vi "Find Center Setup_01282025.vi"(0 "Carrier Tray":T1, 1 "Tray Number":dbl format="%#_13g", 2 "Position":i32, 3 "Assembly Type":string) -> (7 "Assembly Tray Out":T1)   [LabVIEW 2021, in "Assembly Tray.lvclass"]
uses:
  Assembly Tray.lvclass
  Find Tray.ctl
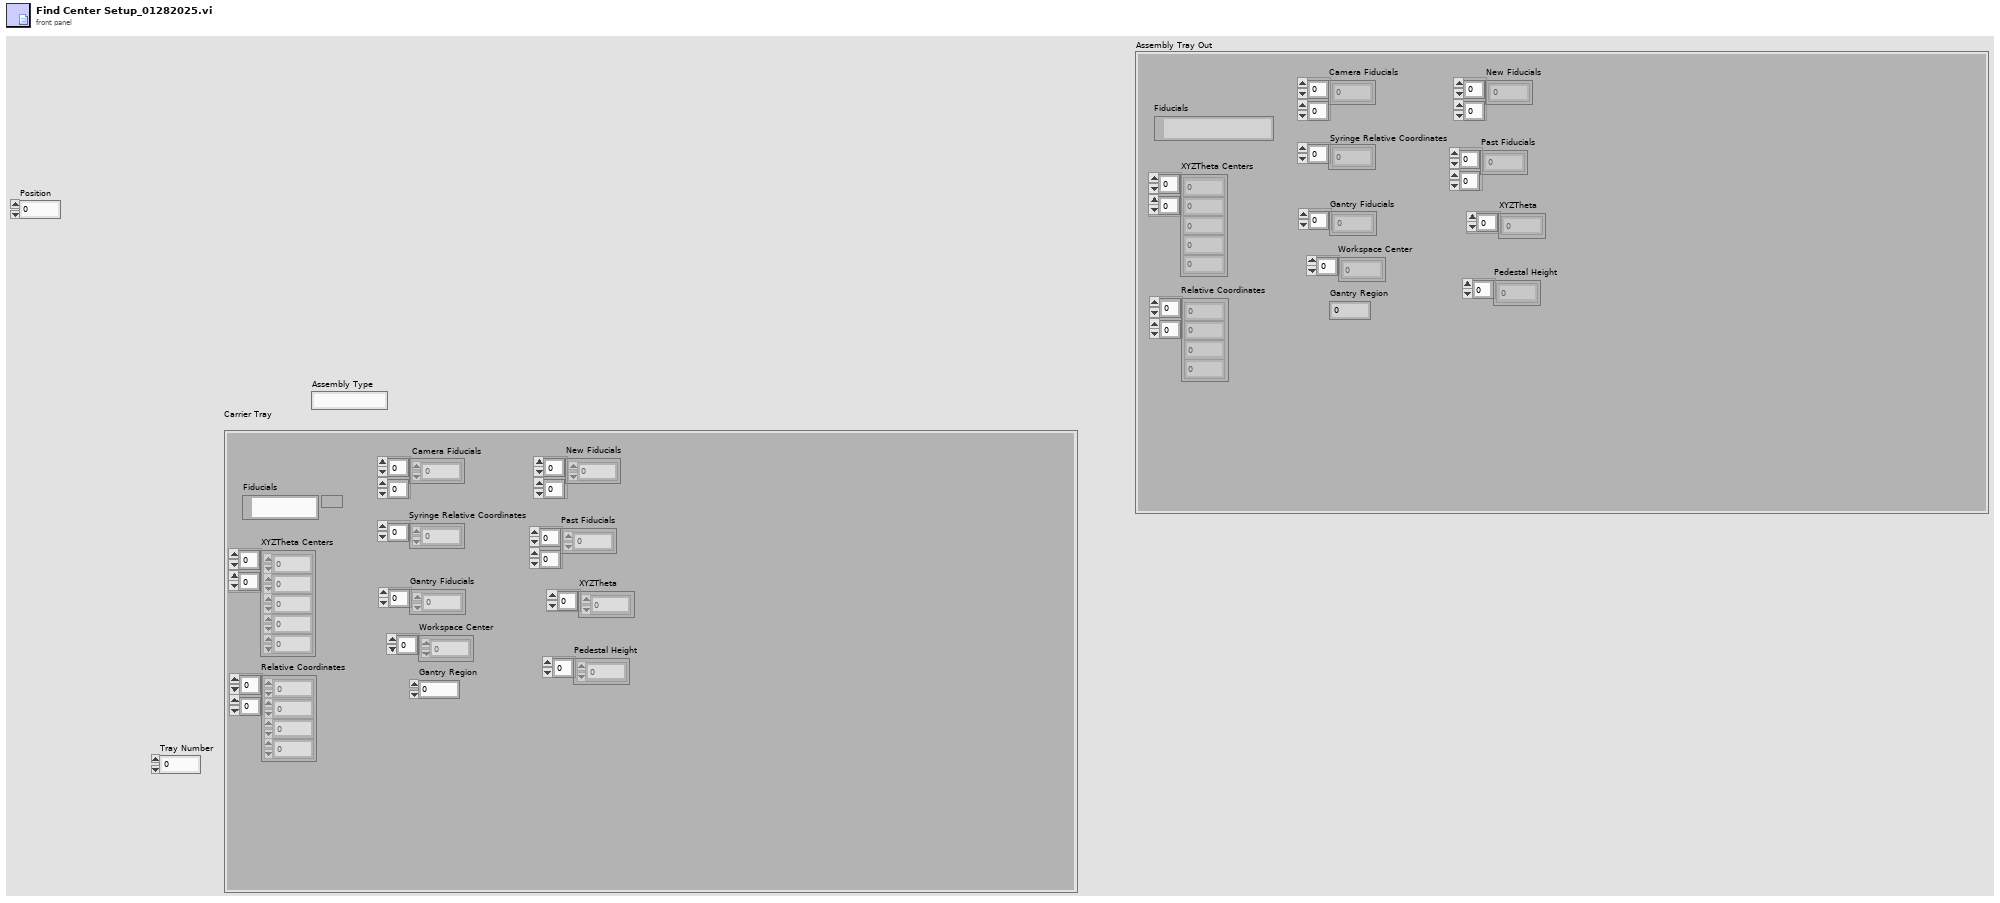
[diagram p1: front panel]
types:
  T1 = typedef "Assembly Tray.lvclass/Find Tray.ctl" = cluster{"Gantry Fiducials":dbl[], "Relative Coordinates":dbl[][], "Camera Fiducials":dbl[][], "XYZTheta Centers":dbl[][], "Workspace Center":dbl[], "Syringe Relative Coordinates":dbl[], "Gantry Region":dbl, "Fiducials":path, "New Fiducials":dbl[][], "Past Fiducials":dbl[][], "XYZTheta":dbl[], "Pedestal Height":dbl[]}
  T2 = typedef "File Paths.ctl" = cluster{"Glue Pattern Folder":path, "Carrier Tray Folder":path, "Pick Up Tool Fixture Folder":path, "Components Folder":path, "Bellows Tool Offset.txt":path, "Pick Up Tool Offset.txt":path, "Dispense Tip Offset.txt":path, "Log Files":path, "Gantry Assembly Map.txt":path, "Syringe and offset map.txt":path, "Controllers Folder":path, "Local dbase config":path}
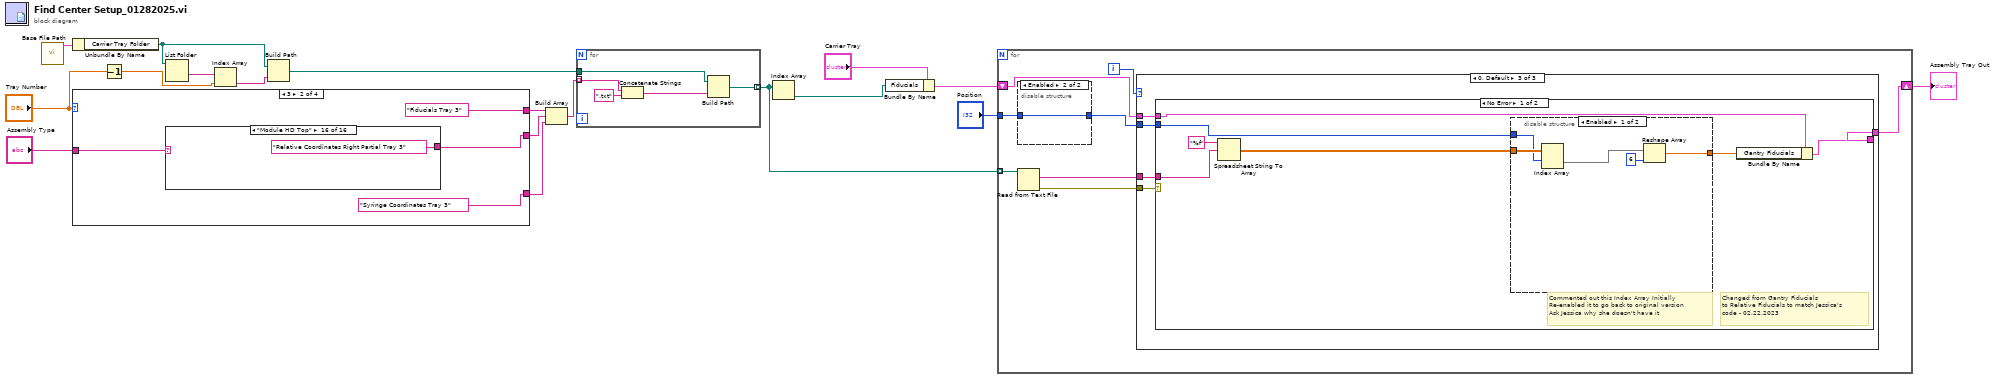
[diagram p0: block diagram]
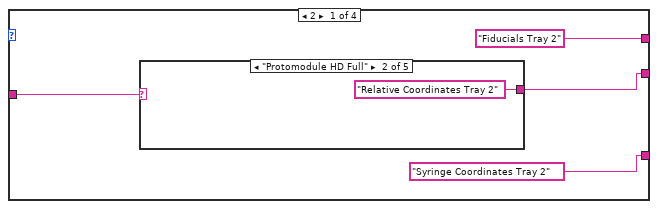
[diagram p2: hidden frame]
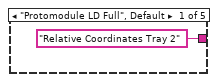
[diagram p3: hidden frame]
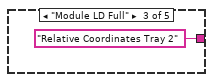
[diagram p4: hidden frame]
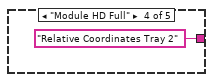
[diagram p5: hidden frame]
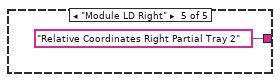
[diagram p6: hidden frame]
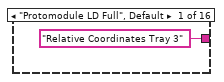
[diagram p7: hidden frame]
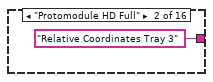
[diagram p8: hidden frame]
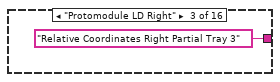
[diagram p9: hidden frame]
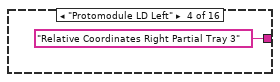
[diagram p10: hidden frame]
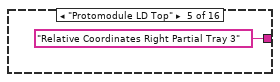
[diagram p11: hidden frame]
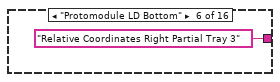
[diagram p12: hidden frame]
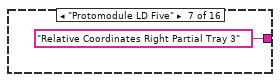
[diagram p13: hidden frame]
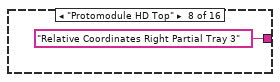
[diagram p14: hidden frame]
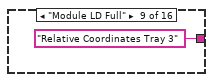
[diagram p15: hidden frame]
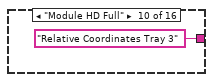
[diagram p16: hidden frame]
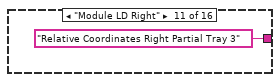
[diagram p17: hidden frame]
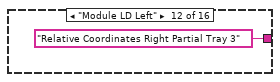
[diagram p18: hidden frame]
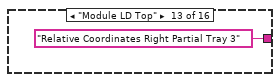
[diagram p19: hidden frame]
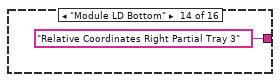
[diagram p20: hidden frame]
diagram:
  n1 = call "Base File Path.vi"() -> ("Paths Out"=w13:T2)  [unwired: 11 in]
  n2 = Unbundle By Name(w13) -> ("Carrier Tray Folder"=w6:path)
  n3 = case shown="3" "Tray Number" {
    tunnel: [w21 w30 w50 w63] -> w9
    tunnel: "Assembly Type" -> [w22 w31 w51 w62]
    tunnel: ["Fiducials Tray 2" ("format string") "Fiducials Tray 3" ("format string") "Fiducials Tray 3" ("format string") "Fiducials" ("format string")] -> w4
    tunnel: ["Syringe Coordinates Tray 2" ("element") "Syringe Coordinates Tray 3" ("element") "Syringe Coordinates Tray 3" ("element") "Syringe Coordinates" ("element")] -> w3
    frame 2 {
      n4 = case shown="\"Protomodule HD Full\"" w22 {
        tunnel: ["Relative Coordinates Tray 2" ("format string") "Relative Coordinates Tray 2" ("format string") "Relative Coordinates Tray 2" ("format string") "Relative Coordinates Tray 2" ("format string") "Relative Coordinates Right Partial Tray 2" ("format string")] -> w21
        frame "Protomodule LD Full", Default {
        }
        frame "Protomodule HD Full" {
        }
        frame "Module LD Full" {
        }
        frame "Module HD Full" {
        }
        frame "Module LD Right" {
        }
      }
    }
    frame 3 {
      n5 = case shown="\"Module HD Top\"" w31 {
        tunnel: ["Relative Coordinates Tray 3" ("format string") "Relative Coordinates Tray 3" ("format string") "Relative Coordinates Right Partial Tray 3" ("format string") "Relative Coordinates Right Partial Tray 3" ("format string") "Relative Coordinates Right Partial Tray 3" ("format string") "Relative Coordinates Right Partial Tray 3" ("format string") "Relative Coordinates Right Partial Tray 3" ("format string") "Relative Coordinates Right Partial Tray 3" ("format string") "Relative Coordinates Tray 3" ("format string") "Relative Coordinates Tray 3" ("format string") "Relative Coordinates Right Partial Tray 3" ("format string") "Relative Coordinates Right Partial Tray 3" ("format string") "Relative Coordinates Right Partial Tray 3" ("format string") "Relative Coordinates Right Partial Tray 3" ("format string") "Relative Coordinates Right Partial Tray 3" ("format string") "Relative Coordinates Right Partial Tray 3" ("format string")] -> w30
        frame "Protomodule LD Full", Default {
        }
        frame "Protomodule HD Full" {
        }
        frame "Protomodule LD Right" {
        }
        frame "Protomodule LD Left" {
        }
        frame "Protomodule LD Top" {
        }
        frame "Protomodule LD Bottom" {
        }
        frame "Protomodule LD Five" {
        }
        frame "Protomodule HD Top" {
        }
        frame "Module LD Full" {
        }
        frame "Module HD Full" {
        }
        frame "Module LD Right" {
        }
        frame "Module LD Left" {
        }
        frame "Module LD Top" {
        }
        frame "Module LD Bottom" {
        }
        frame "Module LD Five" {
        }
        frame "Module HD Top" {
        }
      }
    }
    frame 4 {
      n6 = case shown="\"Module LD Right\"" w51 {
        tunnel: ["Relative Coordinates Tray 3" ("format string") "Relative Coordinates Tray 3" ("format string") "Relative Coordinates Right Partial Tray 3" ("format string") "Relative Coordinates Right Partial Tray 3" ("format string") "Relative Coordinates Tray 3" ("format string") "Relative Coordinates Tray 3" ("format string") "Relative Coordinates Right Partial Tray 4" ("format string") "Relative Coordinates Right Partial Tray 3" ("format string")] -> w50
        frame "Protomodule LD Full", Default {
        }
        frame "Protomodule HD Full" {
        }
        frame "Protomodule LD Right" {
        }
        frame "Protomodule LD Left" {
        }
        frame "Module LD Full" {
        }
        frame "Module HD Full" {
        }
        frame "Module LD Right" {
        }
        frame "Module LD Left" {
        }
      }
    }
    frame 1, Default {
      n7 = case shown="\"Module LD Right\"" w62 {
        tunnel: ["Relative Coordinates" ("format string") "Relative Coordinates" ("format string") "Relative Coordinates Right Partial" ("format string")] -> w63
        frame "Protomodule LD Full", Default {
        }
        frame "Module LD Full" {
        }
        frame "Module LD Right" {
        }
      }
    }
  }
  n8 = Decrement(x="Tray Number") -> (x-1=w11:dbl)
  n9 = List Folder(path=w6) -> (folder names=w15:string[])  [unwired: 3 in, 3 out]
  n10 = Index Array "Index Array"(array=w15, index=w11) -> (element=w14:string)
  n11 = Build Path(base path=w6, name or relative path=w14) -> (appended path=w7:path)
  n12 = Build Array(w4, w9, w3) -> (w16:string[])
  n13 = for {
    tunnel: w16 -> [w70] mode=indexing
    tunnel: w7 -> [w71]
    tunnel: [w67] -> w8 mode=indexing
    n14 = Concatenate Strings "Concatenate Strings"(w70, ".txt" ("string")) -> (w68:string)
    n15 = Build Path(base path=w71, name or relative path=w68) -> (appended path=w67:path)
  }
  n16 = Index Array "Index Array"(array=w8) -> (element=w17:path)  [unwired: 1 in]
  n17 = Bundle By Name "Bundle By Name"(cluster="Carrier Tray", "Fiducials"=w17) -> (w18:T1)
  n18 = for {
    tunnel: w8 -> [w78] mode=indexing
    shift-right: [w74] -> w12
    shift-left: w18 -> [w75]
    tunnel: "Position" -> [w73]
    i -> [w76]
    n19 = disable-structure shown="Enabled" {
      disable-tunnel: w73 -> [w81 w83]
      disable-tunnel: [w80 w83] -> w72
      frame Disabled {
        n20 = Add(x=1, y=w81) -> (x+y=w80:i32)
      }
      frame Enabled {
      }
    }
    n21 = Read from Text File(file (use dialog)=w78) -> (text=w79:string, error out=w77:errorcluster)  [unwired: 3 in, 2 out]
    n22 = case shown="0, Default" w76 {
      tunnel: w79 -> [w86 w101 w117]
      tunnel: w77 -> [w87 w102 w116]
      tunnel: w75 -> [w85 w103 w115]
      tunnel: [w84 w100 w114] -> w74
      tunnel: w72 -> [_ _ w113]
      frame 1 {
        n23 = case shown="No Error" w87 {
          tunnel: w86 -> [w94 _]
          tunnel: [w92 w97] -> w84
          tunnel: w85 -> [w93 w97]
          frame No Error {
            n24 = Spreadsheet String To Array(format string="%f", spreadsheet string=w94, array type (2D Dbl)=dbl[][] []) -> (array=w91:dbl[][])  [unwired: 1 in]
            n25 = Array Subset(array=w91, index (row)=1 ("length"), index (col)=1 ("index (row)")) -> (w90:dbl[][])  [unwired: 2 in]
            n26 = Bundle By Name(cluster=w93, "Relative Coordinates"=w90) -> (w92:T1)
          }
          frame Error {
            n27 = One Button Dialog(message="Relative Coordinates Not Found") -> (true=w98:bool)  [unwired: 1 in]
            n28 = Stop(stop? (T)=w98) -> ()
          }
        }
      }
      frame 2 {
        n29 = case shown="No Error" w102 {
          tunnel: w101 -> [w107 _]
          tunnel: [w105 w110] -> w100
          tunnel: w103 -> [w106 w110]
          frame No Error {
            n30 = Spreadsheet String To Array(format string="%f", spreadsheet string=w107, array type (2D Dbl)=dbl[] []) -> (array=w104:dbl[])  [unwired: 1 in]
            n31 = Bundle By Name(cluster=w106, "Syringe Relative Coordinates"=w104) -> (w105:T1)
          }
          frame Error {
            n32 = One Button Dialog(message="Syringe Coordinates Not Found") -> (true=w111:bool)  [unwired: 1 in]
            n33 = Stop(stop? (T)=w111) -> ()
          }
        }
      }
      frame 0, Default {
        n34 = case shown="No Error" w116 {
          tunnel: w117 -> [w123 _]
          tunnel: w115 -> [w121 w134]
          tunnel: [w122 w134] -> w114
          tunnel: w113 -> [w118 _]
          frame No Error {
            # "Commented out this Index Array Initially\nRe-enabled it to go back to original version\nAsk Jessica why she doesn't have it"
            # "Changed from Gantry Fiducials\nto Relative Fiducials to match Jessica's \ncode - 02.22.2023"
            n35 = Spreadsheet String To Array(format string="%f", spreadsheet string=w123) -> (array=w119:dbl[][])  [unwired: 2 in]
            n36 = disable-structure shown="Enabled" {
              disable-tunnel: [w129 w130] -> w120
              disable-tunnel: w119 -> [w128 w133]
              disable-tunnel: w118 -> [w125 _]
              frame Enabled {
                n37 = Index Array "Index Array"(array=w128, index (row)=w125) -> (element=w127:dbl[])  [unwired: 1 in]
                n38 = Reshape Array "Reshape Array"(w127, 6 ("dimension size")) -> (w129:dbl[])
              }
              frame Disabled {
                n39 = Delete From Array "Delete From Array"() -> ()  [unwired: 3 in, 2 out]
                n40 = Reshape Array "Reshape Array"(w133, 1 ("dimension size"), 1 ("dimension size")) -> (w130:dbl[][])
              }
            }
            n41 = Bundle By Name "Bundle By Name"(cluster=w121, "Gantry Fiducials"=w120) -> (w122:T1)
          }
          frame Error {
            n42 = One Button Dialog(message="Fiducial Data Not Found\nFind Fiducials Manually") -> ()  [unwired: 1 in, 1 out]
          }
        }
      }
    }
  }
  "Assembly Tray Out" <- w12
